vi "CODMn校准记录.vi"(8 "错误输入（无错误）":errorcluster, 11 "data in":T1) -> (0 "错误输出":errorcluster)   [LabVIEW 2016]
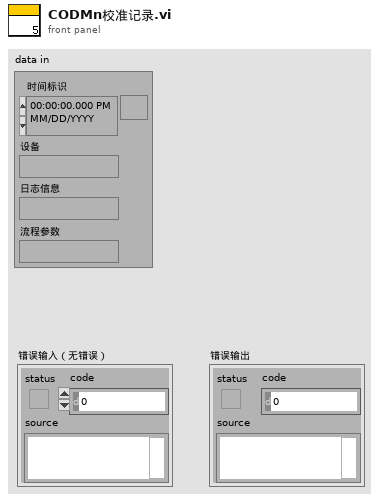
[diagram p1: front panel]
types:
  T1 = cluster{"时间标识":timestamp, "设备":string, "日志信息":string, "流程参数":string}
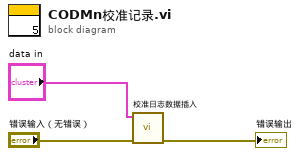
[diagram p0: block diagram]
diagram:
  n1 = call "校准日志数据插入.vi"("data"="data in", "错误输入（无错误）"="错误输入（无错误）") -> ("错误输出"=→"错误输出":errorcluster)  [unwired: 8 in]
